vi "FPGA Main Test.vi"() -> ()   [LabVIEW 2017]
doc: "This VI will will initialize the FPGA VI and then stream analog input data from 4 channels of the 9205."
uses:
  <vilib>/LabVIEW Targets/FPGA/cRIO/shared/nicrio_ModuleControls/nicrio_cRIO-9205_VoltageRange.ctl
  <vilib>/LabVIEW Targets/FPGA/cRIO/shared/nicrio_ModuleControls/nicrio_cRIO-9205_TerminalMode.ctl
  <vilib>/FPGAPlugInAG/cRIO-9067/niLvFpga_Open_cRIO-9067.vi
  <vilib>/rvi/interface/common/dynamic/niFpgaDynamicAddResources.vi
  <vilib>/Utility/error.llb/Error Cluster From Error Code.vi
  <vilib>/rvi/errors/niLvFpgaAdjustHostInterfaceError.vi
  <vilib>/FPGAPlugInAG/Dynamic/niLvFpga_Run_Dynamic.vi
  <vilib>/FPGAPlugInAG/Dynamic/niLvFpga_Close_Dynamic.vi
  <vilib>/rvi/interface/nirviOpenFPGA/nirviOpenFPGA.xnode
  FPGA Bitfiles/cRIONI9205Demo_FPGATarget_FPGAMain_SCyGEa71Jm4.lvbitx
  FPGA Main.vi
  <vilib>/rvi/interface/nirviReadWriteControl/nirviReadWriteControl.xnode
  <vilib>/rvi/interface/nirviMethod/nirviMethod.xnode
  <vilib>/rvi/interface/nirviCloseFPGA/nirviCloseFPGA.xnode
  <vilib>/rvi/interface/Simulation/niFpgaSimulationCallBeginRW.vi
  <vilib>/FPGAPlugInAG/Dynamic/niLvFpga_ReadFifo_Dynamic.vi
  <vilib>/rvi/errors/niLvFpgaMergeErrorWithErrorCode.vi
  NiFpgaLv.dll
panel:
  in  "AI Channel Settings":T3(array[cluster])=[{"Voltage Range"=enum."+/- 10V", "Terminal Mode"=enum."RSE"}, {"Voltage Range"=enum."+/- 10V", "Terminal Mode"=enum."RSE"}, {"Voltage Range"=enum."+/- 10V", "Terminal Mode"=enum."RSE"}, {"Voltage Range"=enum."+/- 10V", "Terminal Mode"=enum."RSE"}]
  out "Data FIFO Full":bool
  out "Voltage Input (V)":dbl[][](graph)
  in  "RT Loop update rate (ms)":u32=100
  out "FPGA error out":errorcluster
  in  "Target Acquisition Rate (Hz)":dbl=10000.0
  out "RT error out":errorcluster
  in  "stop":bool
  # "Overview: Demonstrates data streaming from the 9205 on four analog input channels\nRequirements: LabVIEW FPGA Module, LabVIEW Real-Time Module, NI-RIO\nThis VI will will initialize the FPGA VI and then stream analog input data from 4 channels of the 9205. The 9205's maximum acquisition rate is 250kS/s aggregate. This code is not optimized for speed so you may not be able to achieve this data rate on all controllers.\nInstructions: \n1) Configure Desired AI channel settings and Target Acquisition rate \n2) Run the VI\n3) Modify the RT Loop update rate if desired"
  # "Resource Parameters"
  # "Timing Parameters"
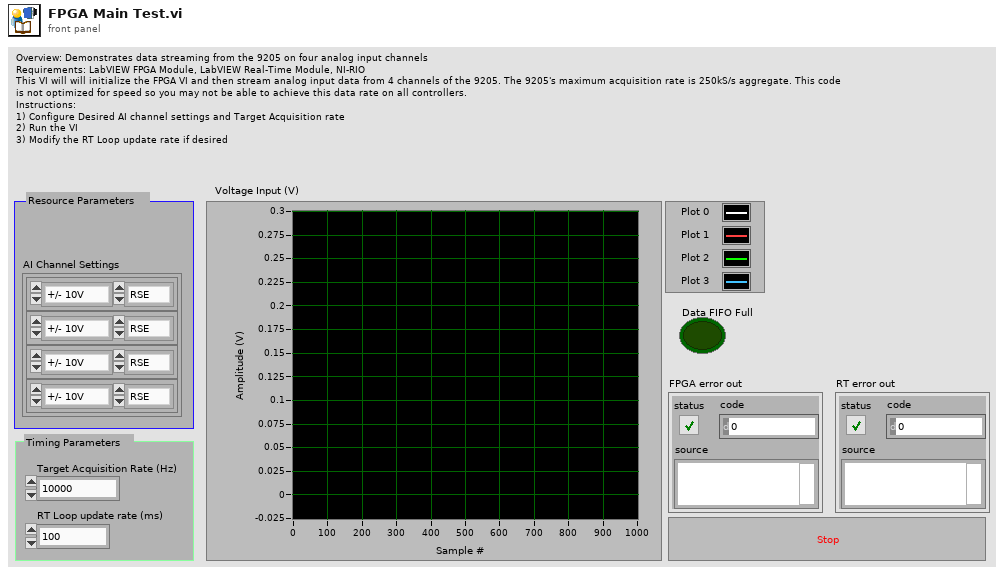
[diagram p1: front panel]
types:
  T1 = typedef "nicrio_cRIO-9205_VoltageRange.ctl" = enum8{"+/- 10V", "+/- 5V", "+/- 1V", "+/- 200mV"}
  T2 = typedef "nicrio_cRIO-9205_TerminalMode.ctl" = enum8{"RSE", "NRSE", "DIFF"}
  T3 = cluster{"Voltage Range":T1, "Terminal Mode":T2}[]
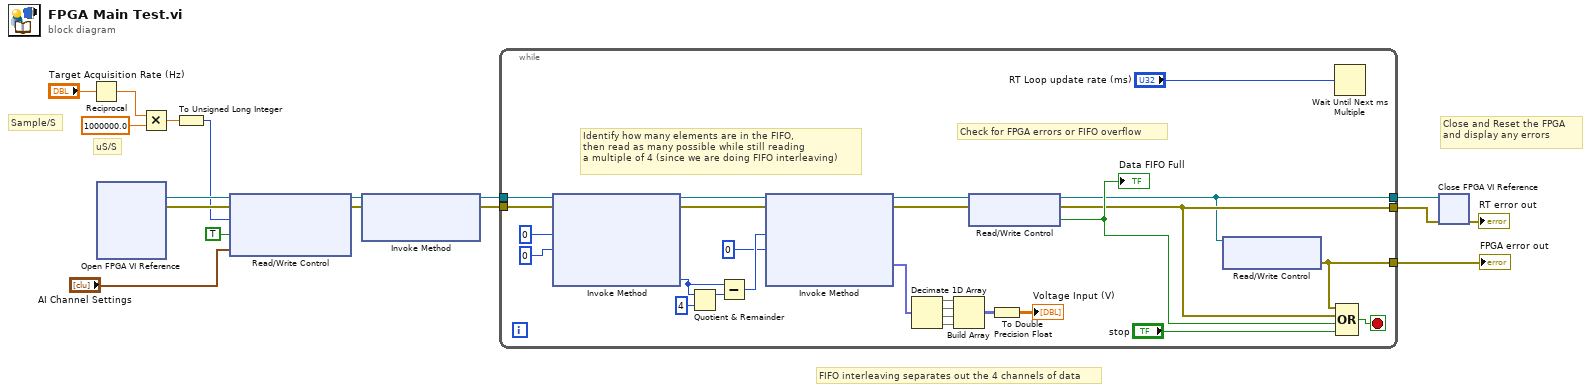
[diagram p0: block diagram]
diagram:
  # "Close and Reset the FPGA\nand display any errors"
  # "FIFO interleaving separates out the 4 channels of data"
  # "Sample/S"
  # "uS/S"
  n1 = Reciprocal(x="Target Acquisition Rate (Hz)") -> (1/x=w12:dbl)
  n2 = xnode "Open FPGA VI Reference"() -> ("FPGA VI Reference Out"=w16:refnum<k20>, "error out"=w15:errorcluster)  [unwired: 2 in]
  n3 = Multiply(x=w12, y=1000000.0) -> (x*y=w10:dbl)
  n4 = To Unsigned Long Integer(number=w10) -> (unsigned 32bit integer=w9:u32)
  n5 = xnode "Read/Write Control"("FPGA VI Reference In"=w16, "error in"=w15, "Loop Rate (uS)"=w9, "Update AI Settings"=TRUE, "AI Channel Settings"="AI Channel Settings") -> ("FPGA VI Reference Out"=w8:refnum<k20>, "error out"=w7:errorcluster)
  n6 = xnode "Invoke Method"("FPGA VI Reference In"=w8, "error in"=w7) -> ("FPGA VI Reference Out"=w6:refnum<k20>, "error out"=w5:errorcluster)  [unwired: 1 in]
  n7 = while {
    tunnel: w6 -> [w30]
    tunnel: w5 -> [w29]
    tunnel: [w20] -> w4
    tunnel: [w19] -> w3
    tunnel: [w18] -> w2
    stop <- w26 stop-if-true
    # "Check for FPGA errors or FIFO overflow"
    # "Identify how many elements are in the FIFO, \nthen read as many possible while still reading\na multiple of 4 (since we are doing FIFO interleaving)"
    n8 = xnode "Invoke Method"("FPGA VI Reference In"=w30, "error in"=w29, "Number of Elements"=u32 0, "Timeout (ms)"=0) -> ("FPGA VI Reference Out"=w41:refnum<k20>, "error out"=w35:errorcluster, "Elements Remaining"=w38:u32)  [unwired: 1 out]
    n9 = Quotient & Remainder(x=w38, y=u32 4) -> (x-y*floor(x/y)=w39:u32)  [unwired: 1 out]
    n10 = Subtract(x=w38, y=w39) -> (x-y=w37:u32)
    n11 = xnode "Invoke Method"("FPGA VI Reference In"=w41, "error in"=w35, "Number of Elements"=w37, "Timeout (ms)"=0) -> ("FPGA VI Reference Out"=w28:refnum<k20>, "error out"=w27:errorcluster, "Data"=w22:fxp<+/-,26,5>[])  [unwired: 1 out]
    n12 = Decimate 1D Array(w22) -> (w31:fxp<+/-,26,5>[], w32:fxp<+/-,26,5>[], w33:fxp<+/-,26,5>[], w34:fxp<+/-,26,5>[])
    n13 = Build Array(w31, w32, w33, w34) -> (w23:fxp<+/-,26,5>[][])
    n14 = xnode "Read/Write Control"("FPGA VI Reference In"=w28, "error in"=w27) -> ("FPGA VI Reference Out"=w19:refnum<k20>, "error out"=w20:errorcluster, "Data FIFO Full"=w21:bool)
    "Data FIFO Full" <- w21
    n15 = To Double Precision Float(number=w23) -> (double precision float=→"Voltage Input (V)":dbl[][])
    n16 = xnode "Read/Write Control"("FPGA VI Reference In"=w19) -> ("FPGA Error Out"=w18:errorcluster)  [unwired: 1 in, 2 out]
    n17 = Wait Until Next ms Multiple(millisecond multiple="RT Loop update rate (ms)") -> ()  [unwired: 1 out]
    n18 = Compound Arithmetic op=OR(w18, w20, w21, "stop") -> (w26:bool)
  }
  "FPGA error out" <- w2
  n19 = xnode "Close FPGA VI Reference"("FPGA VI Reference In"=w3, "error in"=w4) -> ("error out"=→"RT error out":errorcluster)
